vi "Get Current Image.vi"(8 "error in (no error)":errorcluster, 9 "Local Data in":T1, 10 "UI References":T8) -> (0 "error out":errorcluster, 2 "Current Image":string)   [LabVIEW 2024]
uses:
  Controls/RVHR - UI Refs.ctl
  Controls/RVHR - Local Data.ctl
  Controls/Test Cluster.ctl
  Controls/Excluded Information.ctl
  Controls/Language.ctl
  Controls/Device_Type.ctl
  <vilib>/Utility/miscctls.llb/LVRectTypeDef.ctl
  <vilib>/Utility/miscctls.llb/LVBoundsTypeDef.ctl
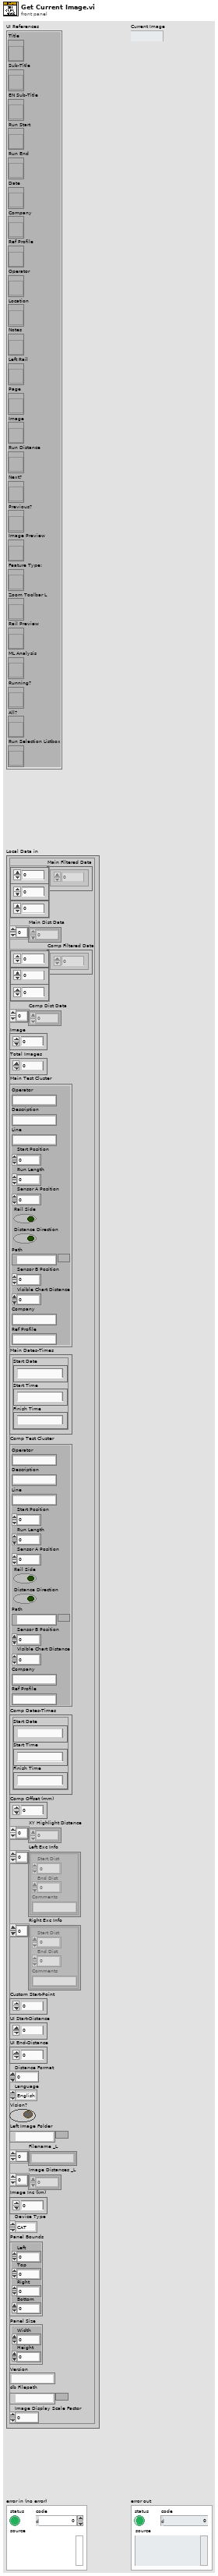
[diagram p1: front panel]
types:
  T1 = typedef "RVHR - Local Data.ctl" = cluster{"Main Filtered Data":dbl[][][], "Main Dist Data":dbl[], "Comp Filtered Data":dbl[][][], "Comp Dist Data":dbl[], "Image":u16, "Total Images":u16, "Main Test Cluster":T2, "Main Dates-Times":cluster{"Start Date":string, "Start Time":string, "Finish Time":string}, "Comp Test Cluster":T2, "Comp Dates-Times":cluster{"Start Date":string, "Start Time":string, "Finish Time":string}, "Comp Offset (mm)":i64, "XY Highlight Distance":dbl[], "Left Exc Info":T3[], "Right Exc Info":T3[], "Custom Start-Point":dbl, "UI Start-Distance":dbl, "UI End-Distance":dbl, "Distance Format":u8, "Language":T4, "Vision?":bool, "Left Image Folder":path, "Filename _L":string[], "Image Distances _L":dbl[], "Image Inc (km)":dbl, "Device Type":T5, "Panel Bounds":T6, "Panel Size":T7, "Version":string, "db Filepath":path, "Image Display Scale Factor":dbl}
  T2 = typedef "Test Cluster.ctl" = cluster{"Operator":string, "Description":string, "Line":string, "Start Position":dbl, "Run Length":dbl, "Sensor A Position":dbl, "Rail Side":bool, "Distance Direction":bool, "Path":path, "Sensor B Position":dbl, "Visible Chart Distance":dbl, "Company":string, "Ref Profile":string}
  T3 = typedef "Excluded Information.ctl" = cluster{"Start Dist":dbl, "End Dist":dbl, "Comments":string}
  T4 = typedef "Language.ctl" = enum16{"English", "Chinese", "German"}
  T5 = typedef "Device_Type.ctl" = enum16{"CAT", "Bi-CAT", "YRCA", "RCA", "RV-HR", "TV-HR"}
  T6 = typedef "LVRectTypeDef.ctl" = cluster{"Left":i16, "Top":i16, "Right":i16, "Bottom":i16}
  T7 = typedef "LVBoundsTypeDef.ctl" = cluster{"Width":u32, "Height":u32}
  T8 = typedef "RVHR - UI Refs.ctl" = cluster{"Title":refnum<vi>, "Sub-Title":refnum<vi>, "EN Sub-Title":refnum<vi>, "Run Start":refnum<vi>, "Run End":refnum<vi>, "Date":refnum<vi>, "Company":refnum<vi>, "Ref Profile":refnum<vi>, "Operator":refnum<vi>, "Location":refnum<vi>, "Notes":refnum<vi>, "Left Rail":refnum<vi>, "Page":refnum<vi>, "Image":refnum<vi>, "Run Distance":refnum<vi>, "Next?":refnum<vi>, "Previous?":refnum<vi>, "Image Preview":refnum<vi>, "Feature Type:":refnum<vi>, "Zoom Toolbar L":refnum<vi>, "Rail Preview":refnum<vi>, "ML Analysis":refnum<vi>, "Running?":refnum<vi>, "All?":refnum<vi>, "Run Selection Listbox":refnum<vi>}
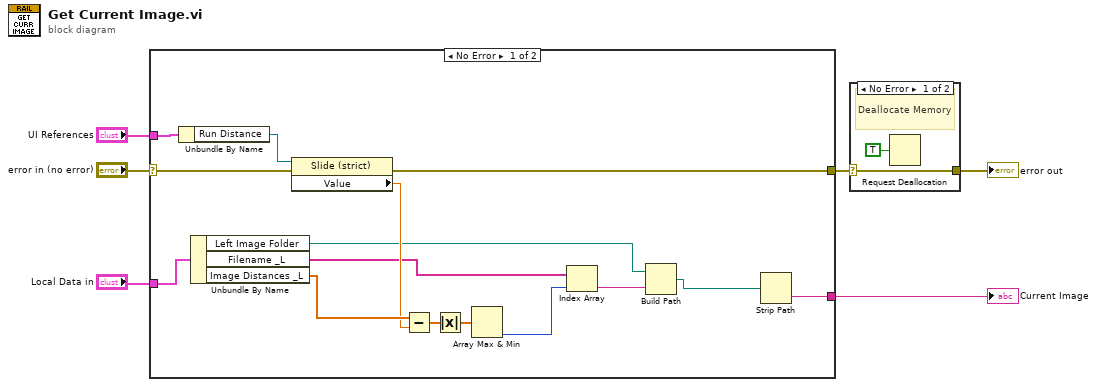
[diagram p0: block diagram]
diagram:
  n1 = case shown="No Error" "error in (no error)" {
    selector: "error in (no error)" -> [w7 w22]
    tunnel: [w18 w22] -> w2
    tunnel: "UI References" -> [w16 _]
    tunnel: [w13 _] -> w5
    tunnel: "Local Data in" -> [w8 _]
    frame No Error {
      n2 = Unbundle By Name(w16) -> ("Run Distance"=w17:refnum<vi>)
      n3 = Unbundle By Name(w8) -> ("Left Image Folder"=w9:path, "Filename _L"=w10:string[], "Image Distances _L"=w20:dbl[])
      n4 = property class="Slide (strict)"(reference=w17, error in=w7) -> (error out=w18:errorcluster, "Value"=w19:dbl)  [unwired: 1 out]
      n5 = Subtract(x=w20, y=w19) -> (x-y=w15:dbl[])
      n6 = Absolute Value(x=w15) -> (abs(x)=w14:dbl[])
      n7 = Array Max & Min(array=w14) -> (min index (indices)=w21:i32)  [unwired: 3 out]
      n8 = Index Array(array=w10, index=w21) -> (element=w11:string)
      n9 = Build Path(base path=w9, name or relative path=w11) -> (appended path=w12:path)
      n10 = Strip Path(path=w12) -> (name=w13:string)  [unwired: 1 out]
    }
    frame Error {
    }
  }
  "Current Image" <- w5
  n11 = case shown="No Error" w2 {
    selector: w2 -> [w23 w25]
    tunnel: [w23 w25] -> w1
    frame No Error {
      # "Deallocate Memory"
      n12 = Request Deallocation(TRUE ("flag")) -> ()
    }
    frame Error {
    }
  }
  "error out" <- w1
